vi "SUB_TelnetLogIN_full.vi"() -> (2 "telnet connection":T1, 3 "Pass ?":bool, 4 "data out":string)   [LabVIEW 2011]
doc: "The Telnet Line Client VI uses the Telnet VIs to simulate a simple Telnet Window."
uses:
  <vilib>/addons/internet/telnet/telnet.llb/Telnet Session.ctl
  Instance           4 28Saved   SUB_TelnetLogIN_full .vi
  Instance           9 28Saved   SUB_TelnetLogIN_full .vi
  Instance           8 28Saved   SUB_TelnetLogIN_full .vi
  <vilib>/addons/internet/NI_InternetTK_Core_VIs.lvlib
panel:
  out "Numeric":i32
  out "KEYWORD2":string
  out "KEYWORD1":string
  out "sec":dbl
  out "begin time":u32
  out "MSG OUT":string
  out "telnet path":string
  out "Setting OK?":bool
  out "TelnetPassword":string
  out "Telnet ID":string
  out "TELNET-IP":string
  out "text":string
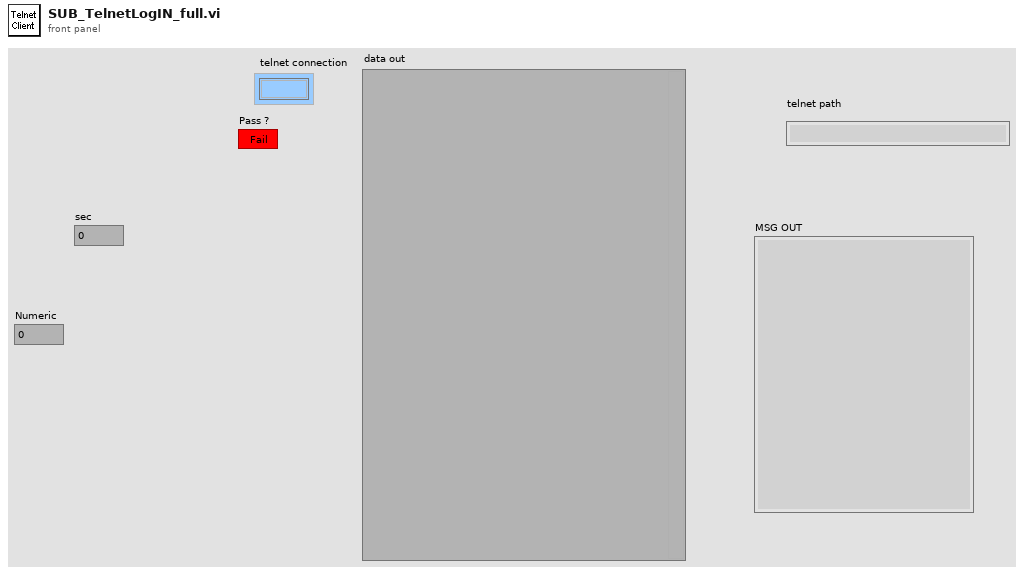
[diagram p1: front panel]
types:
  T1 = typedef "Telnet Session.ctl" = refnum<k1>
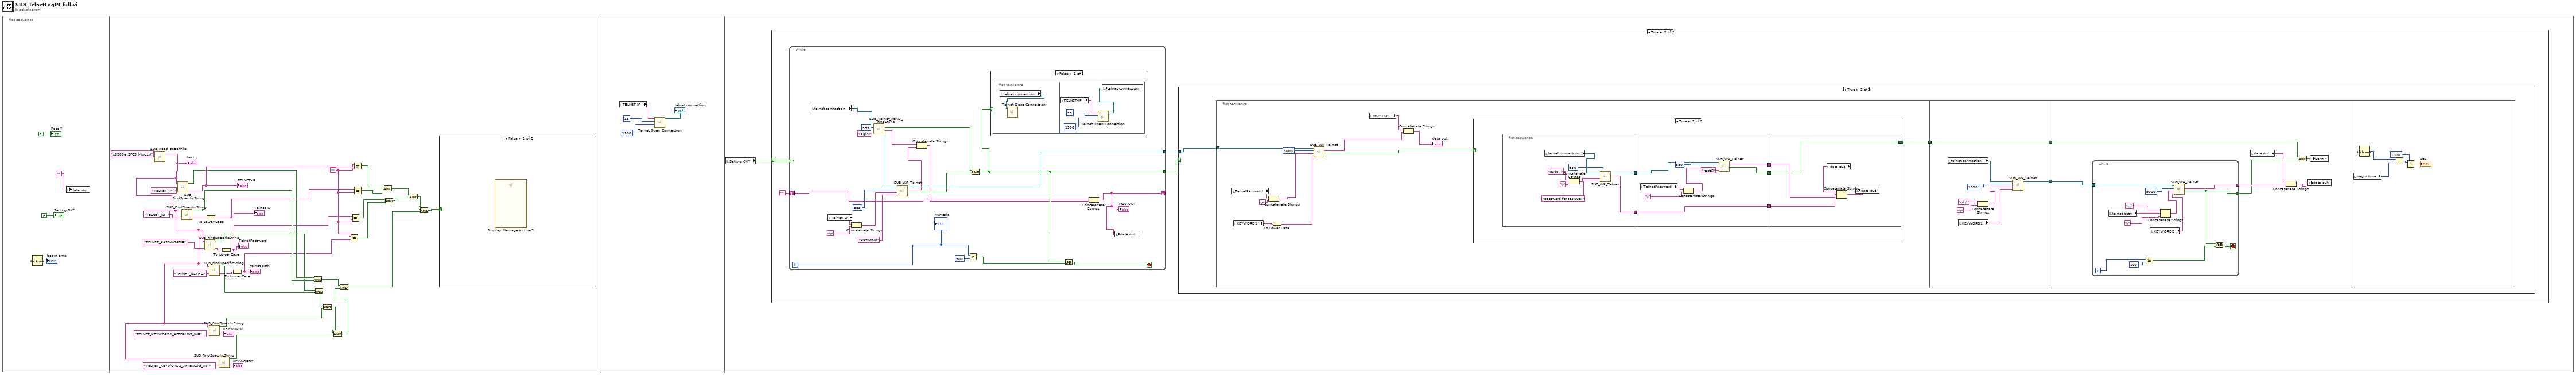
[diagram p0: block diagram]
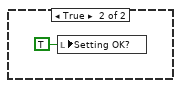
[diagram p2: hidden frame]
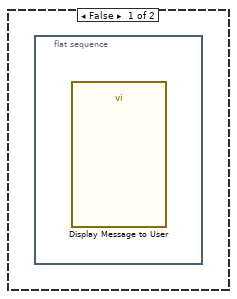
[diagram p5: hidden frame]
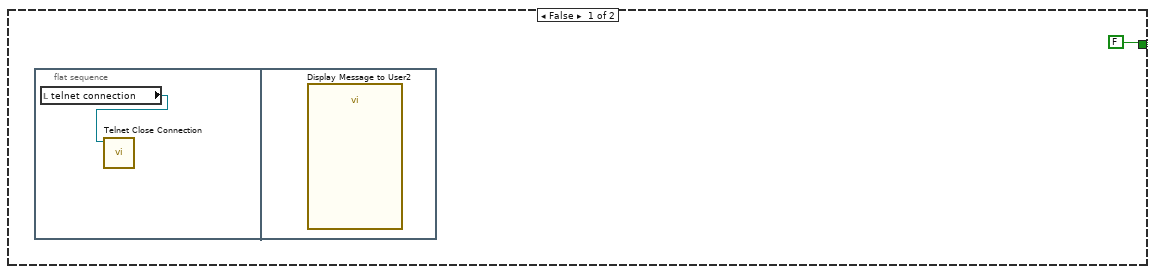
[diagram p6: hidden frame]
diagram:
  n1 = flat-sequence {
    frame #0 {
      n2 = Tick Count (ms)() -> (millisecond timer value=→"begin time":u32)
      n3 = local write "data out"("") -> ()
      "Pass ?" <- FALSE
      "Setting OK?" <- FALSE
    }
    frame #1 {
      w35 = ""
      n4 = call "SUB_Read_specifFile.vi"("name or relative path"="s8300e_SFCS_Misc.txt") -> ("text"=w9:string)  [unwired: 1 in, 1 out]
      "text" <- w9
      n5 = call "SUB_FindSpecificString.vi"("Find this String"="TELNET_IP=", "String data"=w9) -> ("before \"; \" string"=w36:string, "Found"=w34:bool)  [unwired: 2 in]
      "TELNET-IP" <- w36
      n6 = call "SUB_FindSpecificString.vi"("Find this String"="TELNET_ID=" ("string"), "String data"=w9) -> ("before \"; \" string"=w20:string, "Found"=w33:bool)  [unwired: 2 in]
      n7 = call "SUB_FindSpecificString.vi"("Find this String"="TELNET_PASSWORD=", "String data"=w9) -> ("before \"; \" string"=w18:string, "Found"=w32:bool)  [unwired: 2 in]
      n8 = To Lower Case(string=w20) -> (all lower case string=w19:string)
      "Telnet ID" <- w19
      n9 = call "SUB_FindSpecificString.vi"("Find this String"="TELNET_PATH=", "String data"=w9) -> ("before \"; \" string"=w16:string, "Found"=w31:bool)  [unwired: 2 in]
      n10 = call "SUB_FindSpecificString.vi"("Find this String"="TELNET_KEYWORD1_AFTERLOG_IN=", "String data"=w9) -> ("before \"; \" string"=→"KEYWORD1":string, "Found"=w11:bool)  [unwired: 2 in]
      n11 = call "SUB_FindSpecificString.vi"("Find this String"="TELNET_KEYWORD2_AFTERLOG_IN=", "String data"=w9) -> ("before \"; \" string"=→"KEYWORD2":string, "Found"=w6:bool)  [unwired: 2 in]
      n12 = To Lower Case(string=w18) -> (all lower case string=w17:string)
      "TelnetPassword" <- w17
      n13 = To Lower Case(string=w16) -> (all lower case string=w15:string)
      "telnet path" <- w15
      n14 = And(x=w34, y=w33) -> (x .and. y?=w30:bool)
      n15 = And(x=w32, y=w31) -> (x .and. y?=w12:bool)
      n16 = And(x=w12, y=w11) -> (x .and. y?=w7:bool)
      n17 = And(x=w7, y=w6) -> (x .and. y?=w5:bool)
      n18 = And(x=w30, y=w5) -> (x .and. y?=w22:bool)
      n19 = Not Equal?(x=w35, y=w15) -> (x != y?=w24:bool)
      n20 = Not Equal?(x=w17, y=w35) -> (x != y?=w25:bool)
      n21 = Not Equal?(x=w36, y=w35) -> (x != y?=w27:bool)
      n22 = Not Equal?(x=w19, y=w35) -> (x != y?=w26:bool)
      n23 = And(x=w27, y=w26) -> (x .and. y?=w29:bool)
      n24 = And(x=w25, y=w24) -> (x .and. y?=w28:bool)
      n25 = And(x=w29, y=w28) -> (x .and. y?=w23:bool)
      n26 = And(x=w23, y=w22) -> (x .and. y?=w21:bool)
      n27 = case shown="False" w21 {
        frame False {
          n28 = call "Display Message to User3"() -> ()  [unwired: 10 in, 2 out]
        }
        frame True {
          n29 = local write "Setting OK?"(TRUE ("Setting OK?")) -> ()
        }
      }
    }
    frame #2 {
      n30 = local read "TELNET-IP"() -> (w46:string)
      n31 = call <vilib>:"Telnet Open Connection.vi"("timeout ms (60000)"=1500, "remote port (23)"=u16 23, "address"=w46) -> ("telnet connection"=→"telnet connection":T1)  [unwired: 7 in, 1 out]
    }
    frame #3 {
      n32 = local read "Setting OK?"() -> (w47:bool)
      n33 = case shown="True" w47 {
        frame False {
        }
        frame True {
          n34 = while {
            tunnel: [w55] -> w50
            tunnel: [w56] -> w49
            shift-right: [w51] -> _
            shift-left: "" -> [w52]
            i -> [w59]
            stop <- w60 stop-if-true
            n35 = local read "telnet connection"() -> (w54:T1)
            n36 = local read "Telnet ID"() -> (w72:string)
            n37 = Concatenate Strings(w72, "\r") -> (w70:string)
            n38 = call "SUB_Telnet_READ_FindString.vi"("Find this String"="login:", "timeout ms"=555, "telnet connection"=w54) -> ("MSG OUT"=w62:string, "Found"=w64:bool, "telnet connection out"=w65:T1)  [unwired: 6 in]
            n39 = call "SUB_WR_Telnet.vi"("Find this String"="Password:", "data in"=w70, "timeout ms"=555, "telnet connection"=w65) -> ("Found"=w63:bool, "msg out"=w61:string, "telnet connection out"=w55:T1)  [unwired: 1 in]
            n40 = Concatenate Strings(w62, w61) -> (w53:string)
            n41 = Greater Or Equal?(x=w59, y=500) -> (x >= y?=w57:bool)
            n42 = And(x=w64, y=w63) -> (x .and. y?=w56:bool)
            n43 = case shown="False" w56 {
              frame False {
                n44 = flat-sequence {
                  frame #0 {
                    n45 = local read "telnet connection"() -> (w73:T1)
                    n46 = call <vilib>:"Telnet Close Connection.vi"("telnet connection"=w73) -> ()  [unwired: 9 in, 2 out]
                  }
                  frame #1 {
                    n47 = local read "TELNET-IP"() -> (w76:string)
                    n48 = call <vilib>:"Telnet Open Connection.vi"("timeout ms (60000)"=1500, "remote port (23)"=u16 23, "address"=w76) -> ("telnet connection"=w77:T1)  [unwired: 7 in, 1 out]
                    n49 = local write "telnet connection"(w77) -> ()
                  }
                }
              }
              frame True {
              }
            }
            n50 = Or(x=w56, y=w57) -> (x .or. y?=w60:bool)
            n51 = Concatenate Strings(w52, w53) -> (w51:string)
            "MSG OUT" <- w51
            n52 = local write "data out"(w51) -> ()
            "Numeric" <- w59
          }
          n53 = case shown="True" w49 {
            tunnel: w50 -> [_ w81]
            frame False {
              n54 = flat-sequence {
                frame #0 {
                  n55 = call "Display Message to User"() -> ()  [unwired: 10 in, 2 out]
                }
              }
            }
            frame True {
              n56 = flat-sequence {
                tunnel: w81 -> [w89]
                tunnel: [w84] -> w80
                tunnel: w80 -> [w131]
                tunnel: [w131] -> w79
                tunnel: [w124] -> w78
                tunnel: w79 -> [w134]
                tunnel: w78 -> [w133]
                frame #0 {
                  n57 = local read "TelnetPassword"() -> (w92:string)
                  n58 = local read "KEYWORD1"() -> (w83:string)
                  n59 = Concatenate Strings(w92, "\r") -> (w87:string)
                  n60 = To Lower Case(string=w83) -> (all lower case string=w82:string)
                  n61 = call "SUB_WR_Telnet.vi"("Find this String"=w82, "data in"=w87, "timeout ms"=3000, "telnet connection"=w89) -> ("Found"=w85:bool, "msg out"=w86:string)  [unwired: 1 in, 1 out]
                  n62 = local read "MSG OUT"() -> (w91:string)
                  n63 = Concatenate Strings(w91, w86) -> (→"data out":string)
                  n64 = case shown="True" w85 {
                    tunnel: [FALSE w97] -> w84
                    frame False {
                      n65 = flat-sequence {
                        frame #0 {
                          n66 = local read "telnet connection"() -> (w95:T1)
                          n67 = call <vilib>:"Telnet Close Connection.vi"("telnet connection"=w95) -> ()  [unwired: 9 in, 2 out]
                        }
                        frame #1 {
                          n68 = call "Display Message to User2"() -> ()  [unwired: 10 in, 2 out]
                        }
                      }
                    }
                    frame True {
                      n69 = flat-sequence {
                        tunnel: [w103] -> w101
                        tunnel: [w102] -> w99
                        tunnel: w101 -> [w118]
                        tunnel: [w118] -> w100
                        tunnel: w99 -> [w117]
                        tunnel: [w111] -> w98
                        tunnel: [w110] -> w96
                        tunnel: w100 -> [w121]
                        tunnel: w98 -> [w120]
                        tunnel: [w119] -> w97
                        tunnel: w96 -> [w119]
                        frame #0 {
                          n70 = local read "telnet connection"() -> (w107:T1)
                          n71 = Concatenate Strings("sudo -i" ("string"), "\r") -> (w106:string)
                          n72 = call "SUB_WR_Telnet.vi"("Find this String"="password for s8300e: ", "data in"=w106, "timeout ms"=850, "telnet connection"=w107) -> ("msg out"=w103:string, "telnet connection out"=w102:T1)  [unwired: 1 in, 1 out]
                        }
                        frame #1 {
                          n73 = local read "TelnetPassword"() -> (w115:string)
                          n74 = Concatenate Strings(w115, "\r") -> (w113:string)
                          n75 = call "SUB_WR_Telnet.vi"("Find this String"="root@", "data in"=w113, "timeout ms"=850, "telnet connection"=w117) -> ("Found"=w110:bool, "msg out"=w111:string)  [unwired: 1 in, 1 out]
                        }
                        frame #2 {
                          n76 = local read "data out"() -> (w123:string)
                          n77 = Concatenate Strings(w123, w121, w120) -> (w122:string)
                          n78 = local write "data out"(w122) -> ()
                        }
                      }
                    }
                  }
                }
                frame #1 {
                  n79 = local read "telnet connection"() -> (w126:T1)
                  n80 = local read "KEYWORD1"() -> (w130:string)
                  n81 = Concatenate Strings("cd / " ("string"), "\r") -> (w129:string)
                  n82 = call "SUB_WR_Telnet.vi"("Find this String"=w130, "data in"=w129, "timeout ms"=1000, "telnet connection"=w126) -> ("telnet connection out"=w124:T1)  [unwired: 1 in, 2 out]
                }
                frame #2 {
                  n83 = while {
                    tunnel: [w146] -> w137
                    tunnel: w133 -> [w144]
                    tunnel: [w142] -> w132
                    i -> [w141]
                    stop <- w143 stop-if-true
                    n84 = local read "telnet path"() -> (w150:string)
                    n85 = Greater Or Equal?(x=w141, y=100) -> (x >= y?=w139:bool)
                    n86 = local read "KEYWORD2"() -> (w145:string)
                    n87 = Concatenate Strings("cd " ("string"), w150, "\r") -> (w147:string)
                    n88 = call "SUB_WR_Telnet.vi"("Find this String"=w145, "data in"=w147, "timeout ms"=5000, "telnet connection"=w144) -> ("Found"=w142:bool, "msg out"=w146:string)  [unwired: 1 in, 1 out]
                    n89 = Or(x=w142, y=w139) -> (x .or. y?=w143:bool)
                  }
                  n90 = local read "data out"() -> (w138:string)
                  n91 = Concatenate Strings(w138, w137) -> (w136:string)
                  n92 = And(x=w134, y=w132) -> (x .and. y?=w135:bool)
                  n93 = local write "data out"(w136) -> ()
                  n94 = local write "Pass ?"(w135) -> ()
                }
                frame #3 {
                  n95 = local read "begin time"() -> (w155:u32)
                  n96 = Tick Count (ms)() -> (millisecond timer value=w156:u32)
                  n97 = Subtract(x=w156, y=w155) -> (x-y=w154:u32)
                  n98 = Divide(x=w154, y=u32 1000) -> (x/y=→"sec":dbl)
                }
              }
            }
          }
        }
      }
    }
  }
